vi "SignalAcqDev.vi"(8 "error in (no error)":errorcluster caption="entrée d'erreur (pas d'erreur)", 10 "Message":cluster{"Message":string, "Data":variant, i32}, 11 "Experiment en entrée":refnum<class "Experiment.lvclass"> caption="DNL_LabVIEW Object in") -> (0 "error out":errorcluster caption="sortie d'erreur", 3 "Experiment en sortie":refnum<class "Experiment.lvclass"> caption="DNL_LabVIEW Object out")   [LabVIEW 2019, in "Experiment.lvclass"]
uses:
  Experiment.lvclass
  Experiment.lvclass/Experiment.ctl
  <userlib>/GenProg/ArrayTo1DI32.vi
  DevicesClass/BaseDevice/Accessor/GetClassEvent.vi
  DevicesClass/BaseDevice/Accessor/GetClassQueue.vi
  DevicesClass/BaseDevice/BaseDevice.lvclass
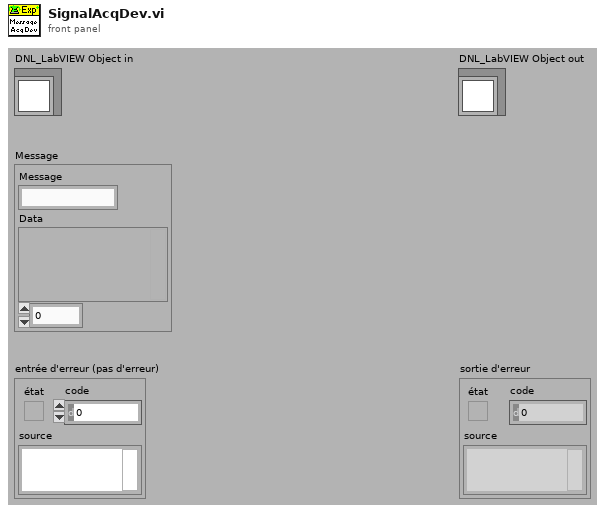
[diagram p1: front panel]
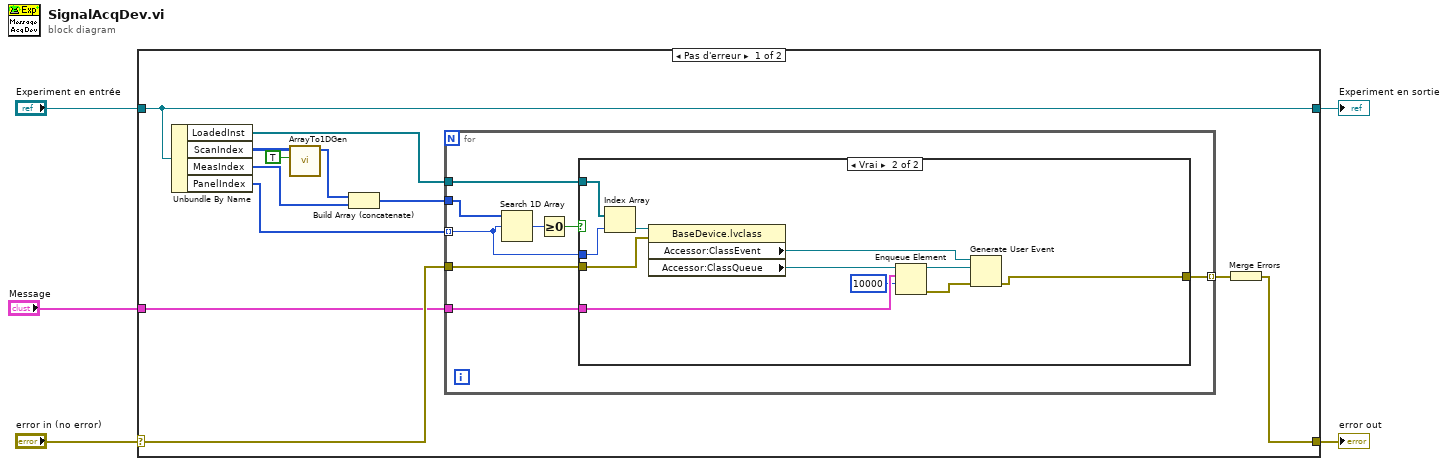
[diagram p0: block diagram]
diagram:
  n1 = case shown="Pas d'erreur" "error in (no error)" {
    selector: "error in (no error)" -> [w9 w39]
    tunnel: [w7 w39] -> w4
    tunnel: [w17 w38] -> w2
    tunnel: "Experiment en entrée" -> [w17 w38]
    tunnel: "Message" -> [w6 _]
    frame No Error {
      n2 = Unbundle By Name(w17) -> ("LoadedInst"=w16:refnum<class "BaseDevice.lvclass">[], "ScanIndex"=w15:i32[][], "MeasIndex"=w13:i32[], "PanelIndex"=w10:i32[])
      n3 = call-poly <userlib>:"ArrayTo1DGen.vi"("DelArrEnd"=TRUE, "tableau"=w15) -> ("Array Out"=w12:i32[])  [unwired: 7 in, 2 out]
      n4 = Build Array (concatenate)(w12, w13) -> (w11:i32[])
      n5 = for {
        tunnel: w16 -> [w22]
        tunnel: w11 -> [w25]
        tunnel: w10 -> [w21] mode=indexing
        tunnel: w9 -> [w20]
        tunnel: [w19] -> w8 mode=indexing
        tunnel: w6 -> [w18]
        n6 = Search 1D Array(1D array=w25, element=w21) -> (index of element=w24:i32)  [unwired: 1 in]
        n7 = Greater Or Equal To 0?(x=w24) -> (x >= 0?=w23:bool)
        n8 = case shown="Vrai" w23 {
          tunnel: w22 -> [_ w37]
          tunnel: w21 -> [_ w36]
          tunnel: w20 -> [w26 w34]
          tunnel: [w26 w30] -> w19
          tunnel: w18 -> [_ w29]
          frame False {
          }
          frame True {
            n9 = Index Array(array=w37, index=w36) -> (element=w35:refnum<class "BaseDevice.lvclass">)
            n10 = property class="BaseDevice.lvclass"(reference=w35, error in=w34) -> ("Accessor:ClassEvent"=w31:refnum<user-event>, "Accessor:ClassQueue"=w28:refnum<queue>)  [unwired: 2 out]
            n11 = Enqueue Element(queue=w28, element=w29, timeout in ms (-1)=10000 ("timeout en ms (-1)")) -> (queue out=w33:refnum<queue>, error out=w32:errorcluster)  [unwired: 1 in, 1 out]
            n12 = Generate User Event(user event=w31, event data cluster=w33, error in=w32) -> (error out=w30:errorcluster)  [unwired: 1 in, 1 out]
          }
        }
      }
      n13 = Merge Errors(w8) -> (w7:errorcluster)
    }
    frame Error {
    }
  }
  "error out" <- w4
  "Experiment en sortie" <- w2
